vi "ROS_Topic_Init.vi"(2 "node":string, 3 "topic":string="/robot/head/command_head_nod") -> (1 "ROS out":T2)   [LabVIEW 2013]
doc: "Initializes a topic and returns a ROS cluster. Required before any read or write call."
uses:
  SubVIs/_ROSControl.ctl
  SubVIs/_ROSDirection.ctl
  _ROSDefinition.vi
panel:
  out "vi name":string
  out "Execution:State":T1(ring)
  out "Already connected?":bool
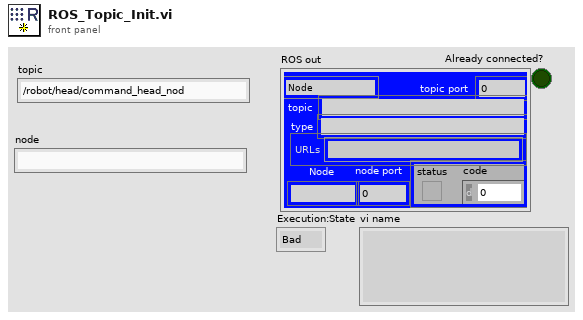
[diagram p1: front panel]
types:
  T1 = enum32{"Bad", "Idle", "Run top level", "Running"}
  T2 = typedef "_ROSControl.ctl" = cluster{"topic port":u16, "Node":string, "topic":string, "type":string, "node port":u32, "error ":errorcluster, "Direction":T3, "APIs":string[]}
  T3 = typedef "_ROSDirection.ctl" = enum16{"Node", "Publisher", "Subscriber", "Service Client"}
  T4 = cluster{"server vi":string, "reference":refnum<vi>, "Description":string[], "Connected":bool}[]
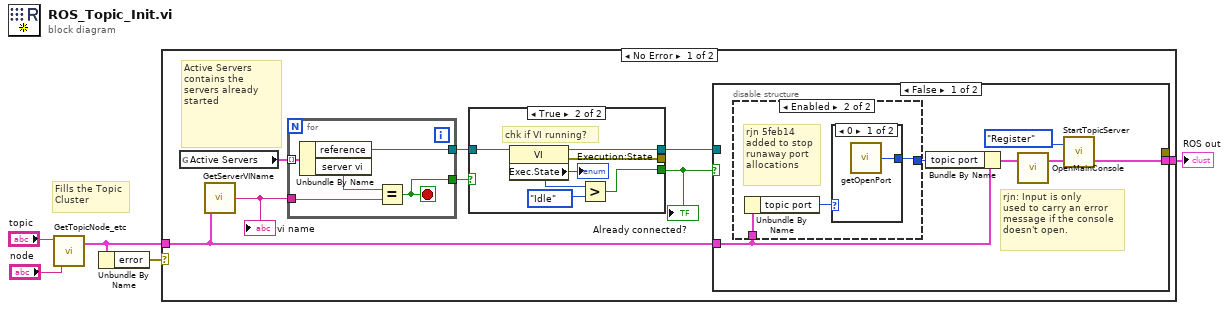
[diagram p0: block diagram]
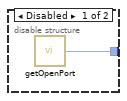
[diagram p2: hidden frame]
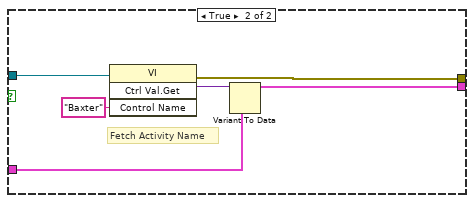
[diagram p4: hidden frame]
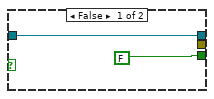
[diagram p5: hidden frame]
diagram:
  # "Fills the Topic\nCluster"
  n1 = call "GetTopicNode_etc.vi"("node"="node", "topic"="topic") -> ("Baxter"=w1:T2)  [unwired: 1 in]
  n2 = Unbundle By Name(w1) -> ("error"=w2:errorcluster)
  n3 = case shown="No Error" w2 {
    tunnel: [w13 w45] -> w5
    tunnel: w1 -> [w6 w45]
    frame No Error {
      # "Active Servers contains the servers already started"
      n4 = global read "_ROSDefinition.vi" "Active Servers"() -> (w12:T4)
      n5 = call "GetServerVIName.vi"("Baxter"=w6) -> ("vi name"=w11:string)
      "vi name" <- w11
      n6 = for {
        tunnel: w12 -> [w44] mode=indexing
        tunnel: w11 -> [w42]
        tunnel: [w41] -> w9
        tunnel: [w40] -> w7
        stop <- w41 stop-if-true
        n7 = Unbundle By Name(w44) -> ("reference"=w40:refnum<vi>, "server vi"=w43:string)
        n8 = Equal?(x=w43, y=w42) -> (x = y?=w41:bool)
      }
      n9 = case shown="True" w9 {
        tunnel: w7 -> [w32 w39]
        tunnel: [FALSE w35] -> w10
        tunnel: [w32 w34] -> w8
        tunnel: [_ w36] -> _
        frame False {
        }
        frame True {
          # "chk if VI running?"
          n10 = property class="VI"(reference=w39) -> (reference out=w34:refnum<vi>, error out=w36:errorcluster, "Exec.State"=w38:T1)  [unwired: 1 in]
          "Execution:State" <- w38
          n11 = Greater?(x=w38, y=T1."Idle") -> (0:w35:bool)
        }
      }
      "Already connected?" <- w10
      n12 = case shown="False" w10 {
        tunnel: [w19 w27] -> w13
        tunnel: w6 -> [w14 w28]
        tunnel: w8 -> [_ w29]
        tunnel: [_ w26] -> _
        frame False {
          # "rjn: Input is only\nused to carry an error \nmessage if the console\ndoesn't open."
          n13 = disable-structure shown="Enabled" {
            disable-tunnel: [w20 w21] -> w16
            disable-tunnel: w14 -> [_ w23]
            frame Disabled {
              n14 = call "getOpenPort.vi"() -> ("port"=w20:u16)
            }
            frame Enabled {
              # "rjn 5feb14\nadded to stop\nrunaway port\nallocations"
              n15 = Unbundle By Name(w23) -> ("topic port"=w22:u16)
              n16 = case shown="0" w22 {
                selector: w22 -> [_ w25]
                tunnel: [w24 w25] -> w21
                frame 0 {
                  n17 = call "getOpenPort.vi"() -> ("port"=w24:u16)
                }
                frame Default {
                }
              }
            }
          }
          n18 = Bundle By Name(cluster=w14, "topic port"=w16) -> (w15:T2)
          n19 = call "OpenMainConsole.vi"("Baxter in"=w15) -> ("Baxter out"=w17:T2)  [unwired: 2 in]
          n20 = call "StartTopicServer.vi"("Baxter in"=w17, "Registration"=enum16{"Register", "Unregister"}."Register") -> ("Baxter out"=w19:T2)  [unwired: 1 in]
        }
        frame True {
          # "Fetch Activity Name"
          n21 = invoke class="VI" method="Ctrl Val.Get"(reference=w29, "Control Name"="Baxter") -> (error out=w26:errorcluster, "Get Control Value Variant"=w31:variant)  [unwired: 2 in, 2 out]
          n22 = Variant To Data(type=w28, Variant=w31) -> (data=w27:T2)  [unwired: 1 in, 1 out]
        }
      }
    }
    frame Error {
    }
  }
  "ROS out" <- w5
